vi "main.vi"() -> ()   [LabVIEW 2015]
uses:
  <vilib>/Utility/error.llb/whitespace.ctl
  <vilib>/MakerHub/LINX/Public/Peripherals/Analog/Analog Read N Chans.vi
  <vilib>/MakerHub/LINX/Public/Peripherals/Digital/Digital Write 1 Chan.vi
  <vilib>/MakerHub/LINX/Private/Local IO/LinxAnalogRead.vi
  <vilib>/MakerHub/LINX/Public/Utilities/Check Channel.vi
  <vilib>/MakerHub/LINX/Public/Peripherals/Digital/Digital Write N Chans.vi
  <vilib>/MakerHub/LINX/Private/Local IO/LinxDigitalWrite.vi
  <vilib>/Instr/_visa.llb/VISA Configure Serial Port (Instr).vi
  <vilib>/MakerHub/LINX/Public/Utilities/Open Serial.vi
  <vilib>/MakerHub/LINX/Private/Utilties/Generate Error.vi
  <vilib>/ptbypt/NI_PtbyPt.lvlib
  <vilib>/MakerHub/LINX/LMH-LINX.lvlib
  Report (lvlib)/Report - CSV/Report - CSV.lvlib
panel:
  out "baocao NG 2":bool
  out "baocao NG 1":bool
  in  "?":T1(tab)=enum."CONTROL & SUPERVISORY"
  in  "Result":i32(listbox)=-1
  in  "Delete table":bool
  out "Form QR ?":bool
  out "Data#":bool
  out "Found?":bool
  out "False Package":dbl
  out "SS3":bool=TRUE
  out "SS2":bool=TRUE
  out "SS1":bool=TRUE
  out "Processing Chart":cluster{dbl, dbl, dbl, dbl, "mean":dbl}(graph)={0.0, 0.0, 0.0, -16.408877733961745, "mean"=-16.408877733961745}
  out "WEIGHT PASS":bool
  out "Calculate\nValue":dbl=88.0
  out "DATA":string="ID: 3\nC/N: c8035\nQuantity: 42\nMass: 1.56\r\nS/N: 1\nC/N: vit dai\nQuantity: 3\nMass: 27\r\n"
  out "QR PASS":bool
  out "Well Package":i32
  out "Measurement\nValue":dbl format="%#.3f"
  in  "zero":bool
  in  "No. \nAccurate":dbl=10.0 format="%#_13g"
  in  "STOP":bool
  in  "Start measurement":bool caption="Manual\nMeasurement"
  out "CTHT1":bool=TRUE
  out "CTHT2":bool=TRUE
  out "Trigger1":bool
  out "Trigger 2":bool
  in  "k/lg bao bi":dbl=7.0 format="%#.3f"
  out "Run Loop":i32=6737
  out "?":T2(plugin-control)
  in  "measurement":dbl=38.0
  in  "calculate":dbl=50.0
  out "S/N":string
  out "C/N":string
  in  "Sensor Channels":u8[](array[numeric])=[0, 1, 2, 3, 4]
  in  "Path save data report":path=path "C:/Data"
  in  "COM Port Controller":refnum<visa-resource-name>="COM12"
  out "Quantity":i32=3
  out "Mass (kg):":dbl=27.0
  out "Tong K/lg (kg)":dbl=88.0
  in  "VISA resource name":refnum<visa-resource-name>="COM10"
  out "Data from HX711 box":i32[](array[numeric])
  out "size array":i32=233
  out "Raw data":dbl
  out "Fine Data":dbl=-16.408877733961745
  in  "zero":dbl=16.408877733961745
  in  "he so calib":dbl=8.552828494462736 format="%#_12g"
  in  "Low factor":cluster{"1":dbl, "2":dbl, "3":dbl}={"1"=177000.0, "2"=222000.0, "3"=-207250.0}
  in  "High Factor":cluster{"1":dbl, "2":dbl, "3":dbl}={"1"=1073000.0, "2"=1137000.0, "3"=703000.0} {"3" format="%#_15f"}
  in  "sample length":i32=100
  in  "No. model\nto Zero":i32=500
  in  "Pulse pin 2":u8=4
  in  "DIR pin 2":u8=3
  out "notifier out":refnum<notifier>
  in  "V-ref-trigger":dbl=0.2 format="%#_13g"
  out "Sensors Chart":T3(graph)={"Voltages[0]"=4.2626953125, "Voltages[1]"=4.27734375, "Voltages[2]"=4.2626953125, "Voltages[3]"=4.2626953125, "Voltages[4]"=4.2578125, "Voltages[5]"=0.0, "Voltages[6]"=0.0, "Voltages[7]"=0.0, "Voltages[8]"=0.0}
  in  "Enable pin 2":u8=2
  in  "Frequency (Hz) 2":u32=1600
  in  "Frequency (Hz)":u32=1600
  in  "Pulse pin":u8=4
  in  "DIR pin":u8=3
  in  "enable pin":u8=2
  in  "File name .csv":string="a"
  in  "Reset model":bool
  in  "button SS 1":bool
  in  "button SS 2":bool
  in  "button SS 3":bool
  in  "button CTHT 1":bool
  in  "button CTHT 2":bool
  out "STT":dbl format="%#_13g"
  out "gat hang 2":bool
  out "gat hang":bool
  out "Done QR":bool
  out "Appear":bool
  # "HÊò THÔìNG KIÊÒM TRA CHÂìT LÝÕòNG ÐOìNG GOìI THUÌNG HAÌNG\n THEO MAÞ QR & ÌKHÔìI LÝÕòNG"
  # "Table Result"
  # "(g)"
  # "(g)"
  # "Sensors"
  # "Control"
  # "Weight Transmit"
  # "Motor1"
  # "Motor2"
  # "Result Image Processing"
  # "Report"
  # "Distance Sensors and Limit Switch"
  # "TEST"
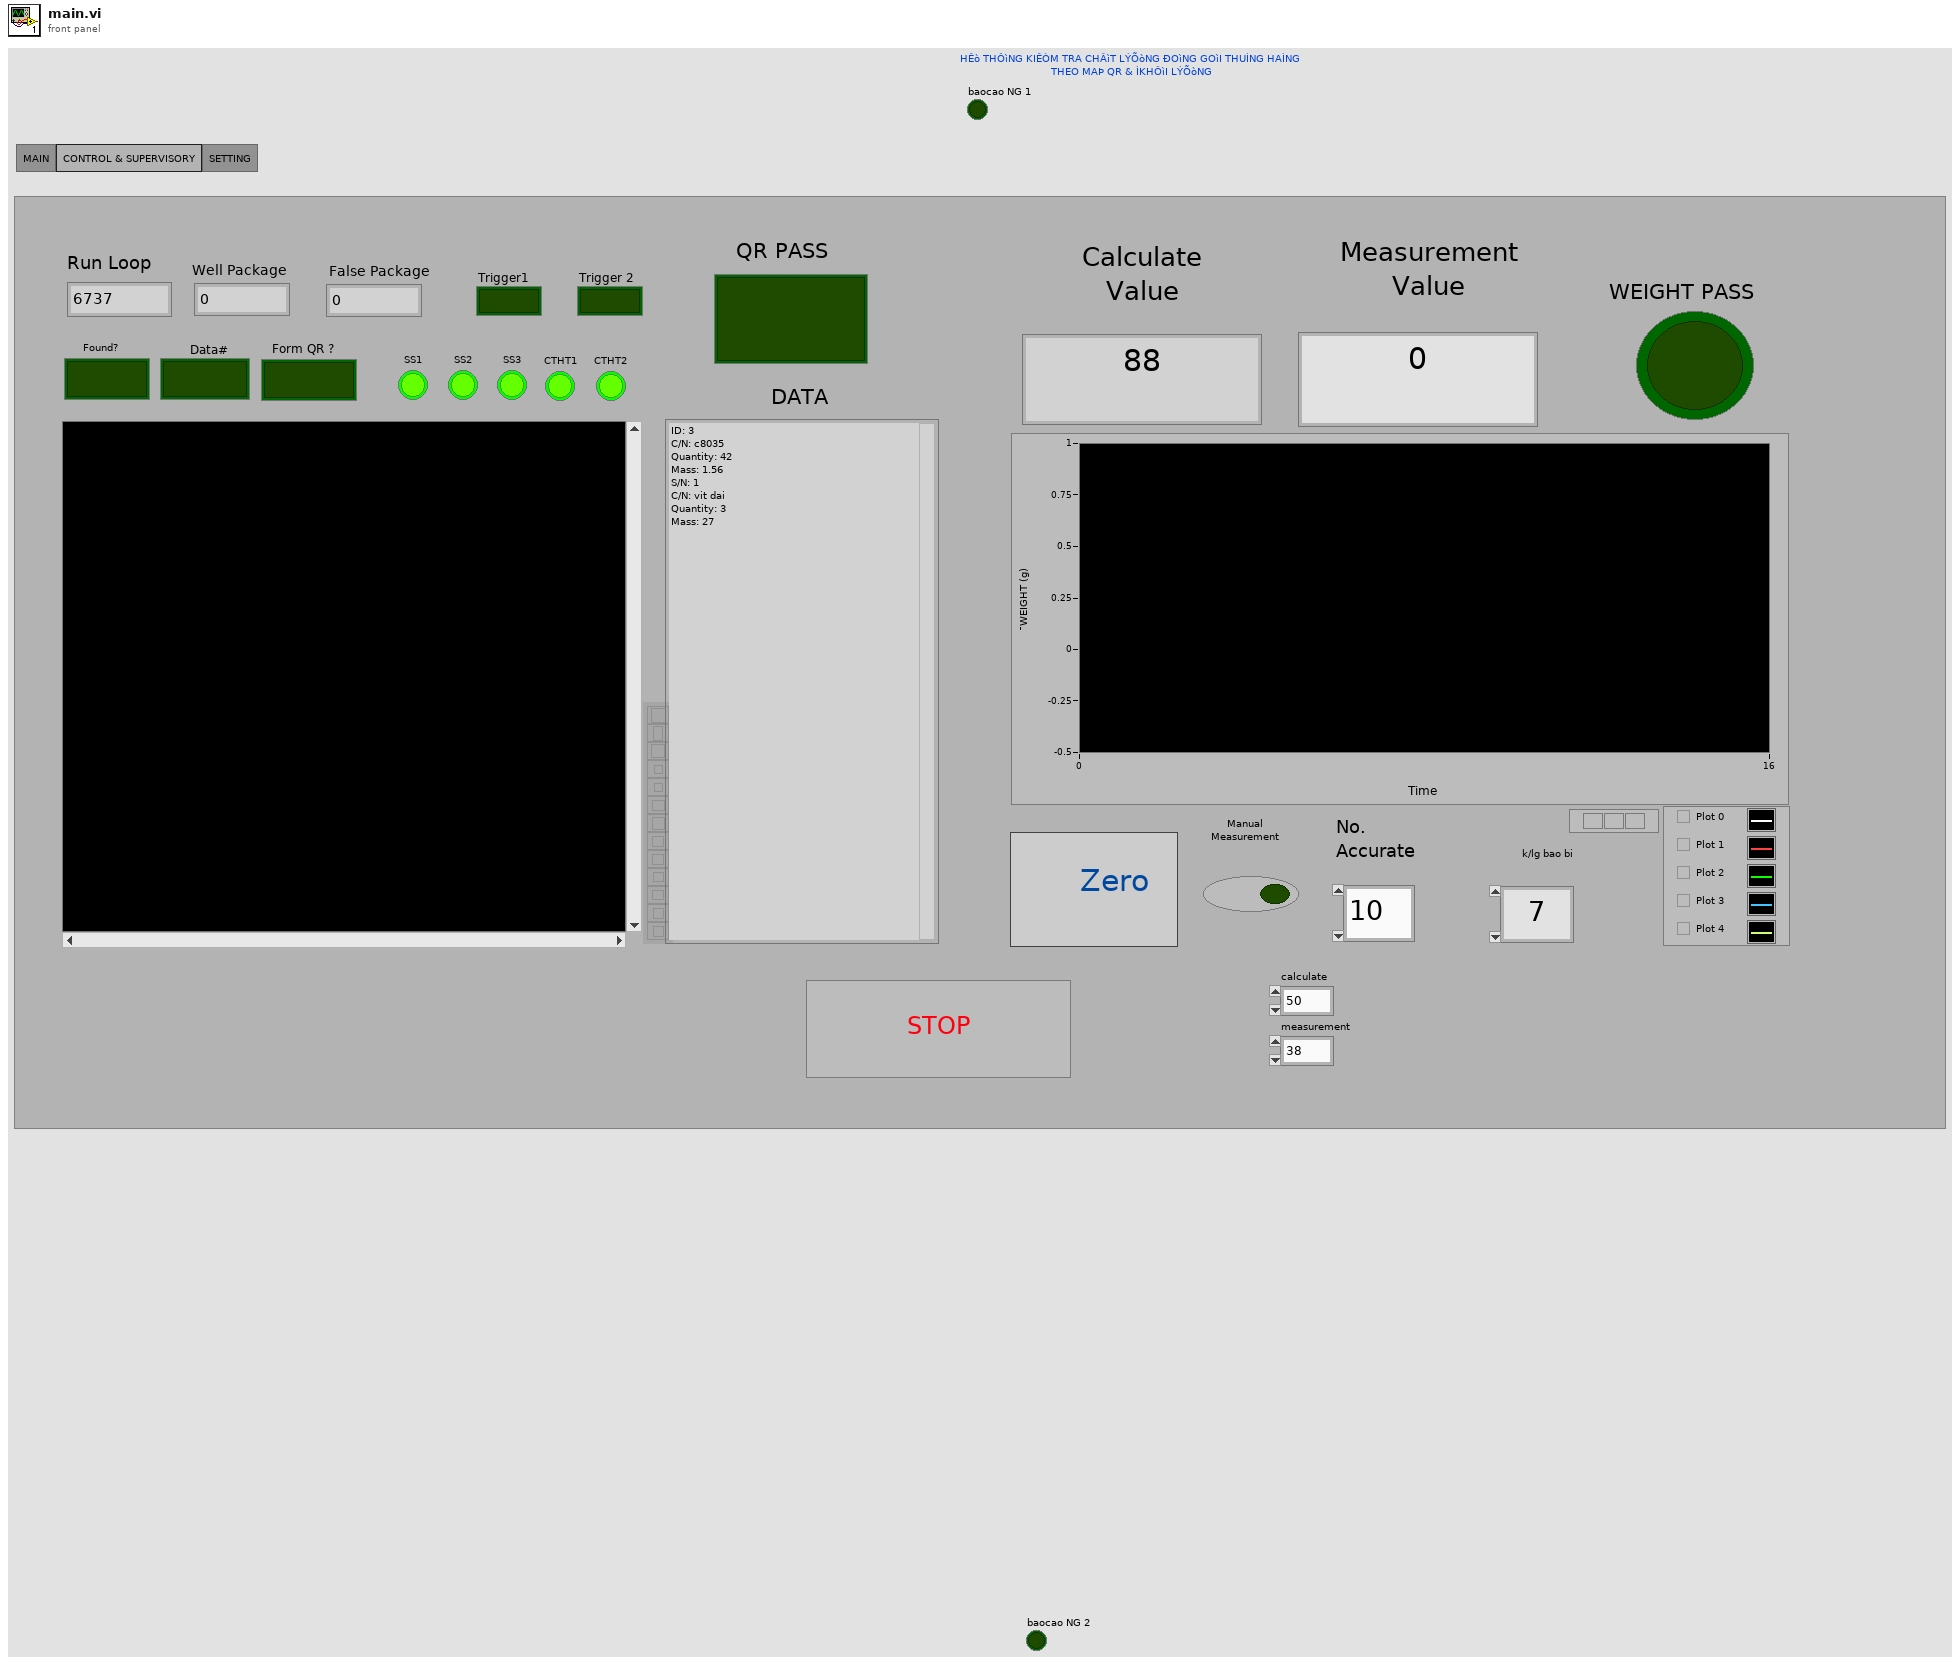
[diagram p1: front panel]
types:
  T1 = enum32{"MAIN", "CONTROL & SUPERVISORY", "SETTING"}
  T2 = typedef "IMAQ Image.ctl" = refnum<image>
  T3 = cluster{"Voltages[0]":dbl, "Voltages[1]":dbl, "Voltages[2]":dbl, "Voltages[3]":dbl, "Voltages[4]":dbl, "Voltages[5]":dbl, "Voltages[6]":dbl, "Voltages[7]":dbl, "Voltages[8]":dbl}
  T4 = cluster{"baud rate":u32, "data bits":u16, "parity":enum16{"None", "Odd", "Even", "Mark", "Space"}, "stop bits":u16, "flow control":u16}
  T5 = typedef "LMH-LINX.lvlib/LINX Ref.ctl" = cluster{"IO":T6, "Interface":T7, "LINX Device Config":T8}
  T6 = typedef "LMH-LINX.lvlib/Platform.ctl" = enum16{"Remote", "Local"}
  T7 = typedef "LMH-LINX.lvlib/Interface.ctl" = enum16{"Serial", "TCP"}
  T8 = typedef "LMH-LINX.lvlib/Device.lvlib/LINX Device Config.ctl" = cluster{"Interface":T7, "COM Port":refnum<visa-resource-name>, "TCP Configuration":T9, "Device Family":u8, "Device ID":u8, "Device Name":string, "TCP Ref":refnum<k5>, "Channels":T10}
  T9 = typedef "LMH-LINX.lvlib/Device.lvlib/TCP Config.ctl" = cluster{"IP Address":string, "Port":u16}
  T10 = typedef "LMH-LINX.lvlib/Channels.ctl" = cluster{"DI":u8[], "DO":u8[], "AI":u8[], "AO":u8[], "PWM":u8[], "QE":u8[], "UART":u8[], "I2C 2":u8[], "SPI":u8[], "CAN":u8[], "Servo":u8[], "AI Ref (V)":dbl, "AI Resolution (Bits)":u8, "AO Ref (V)":dbl, "AO Resolution (Bits)":u8}
  T11 = typedef "whitespace.ctl" = u16
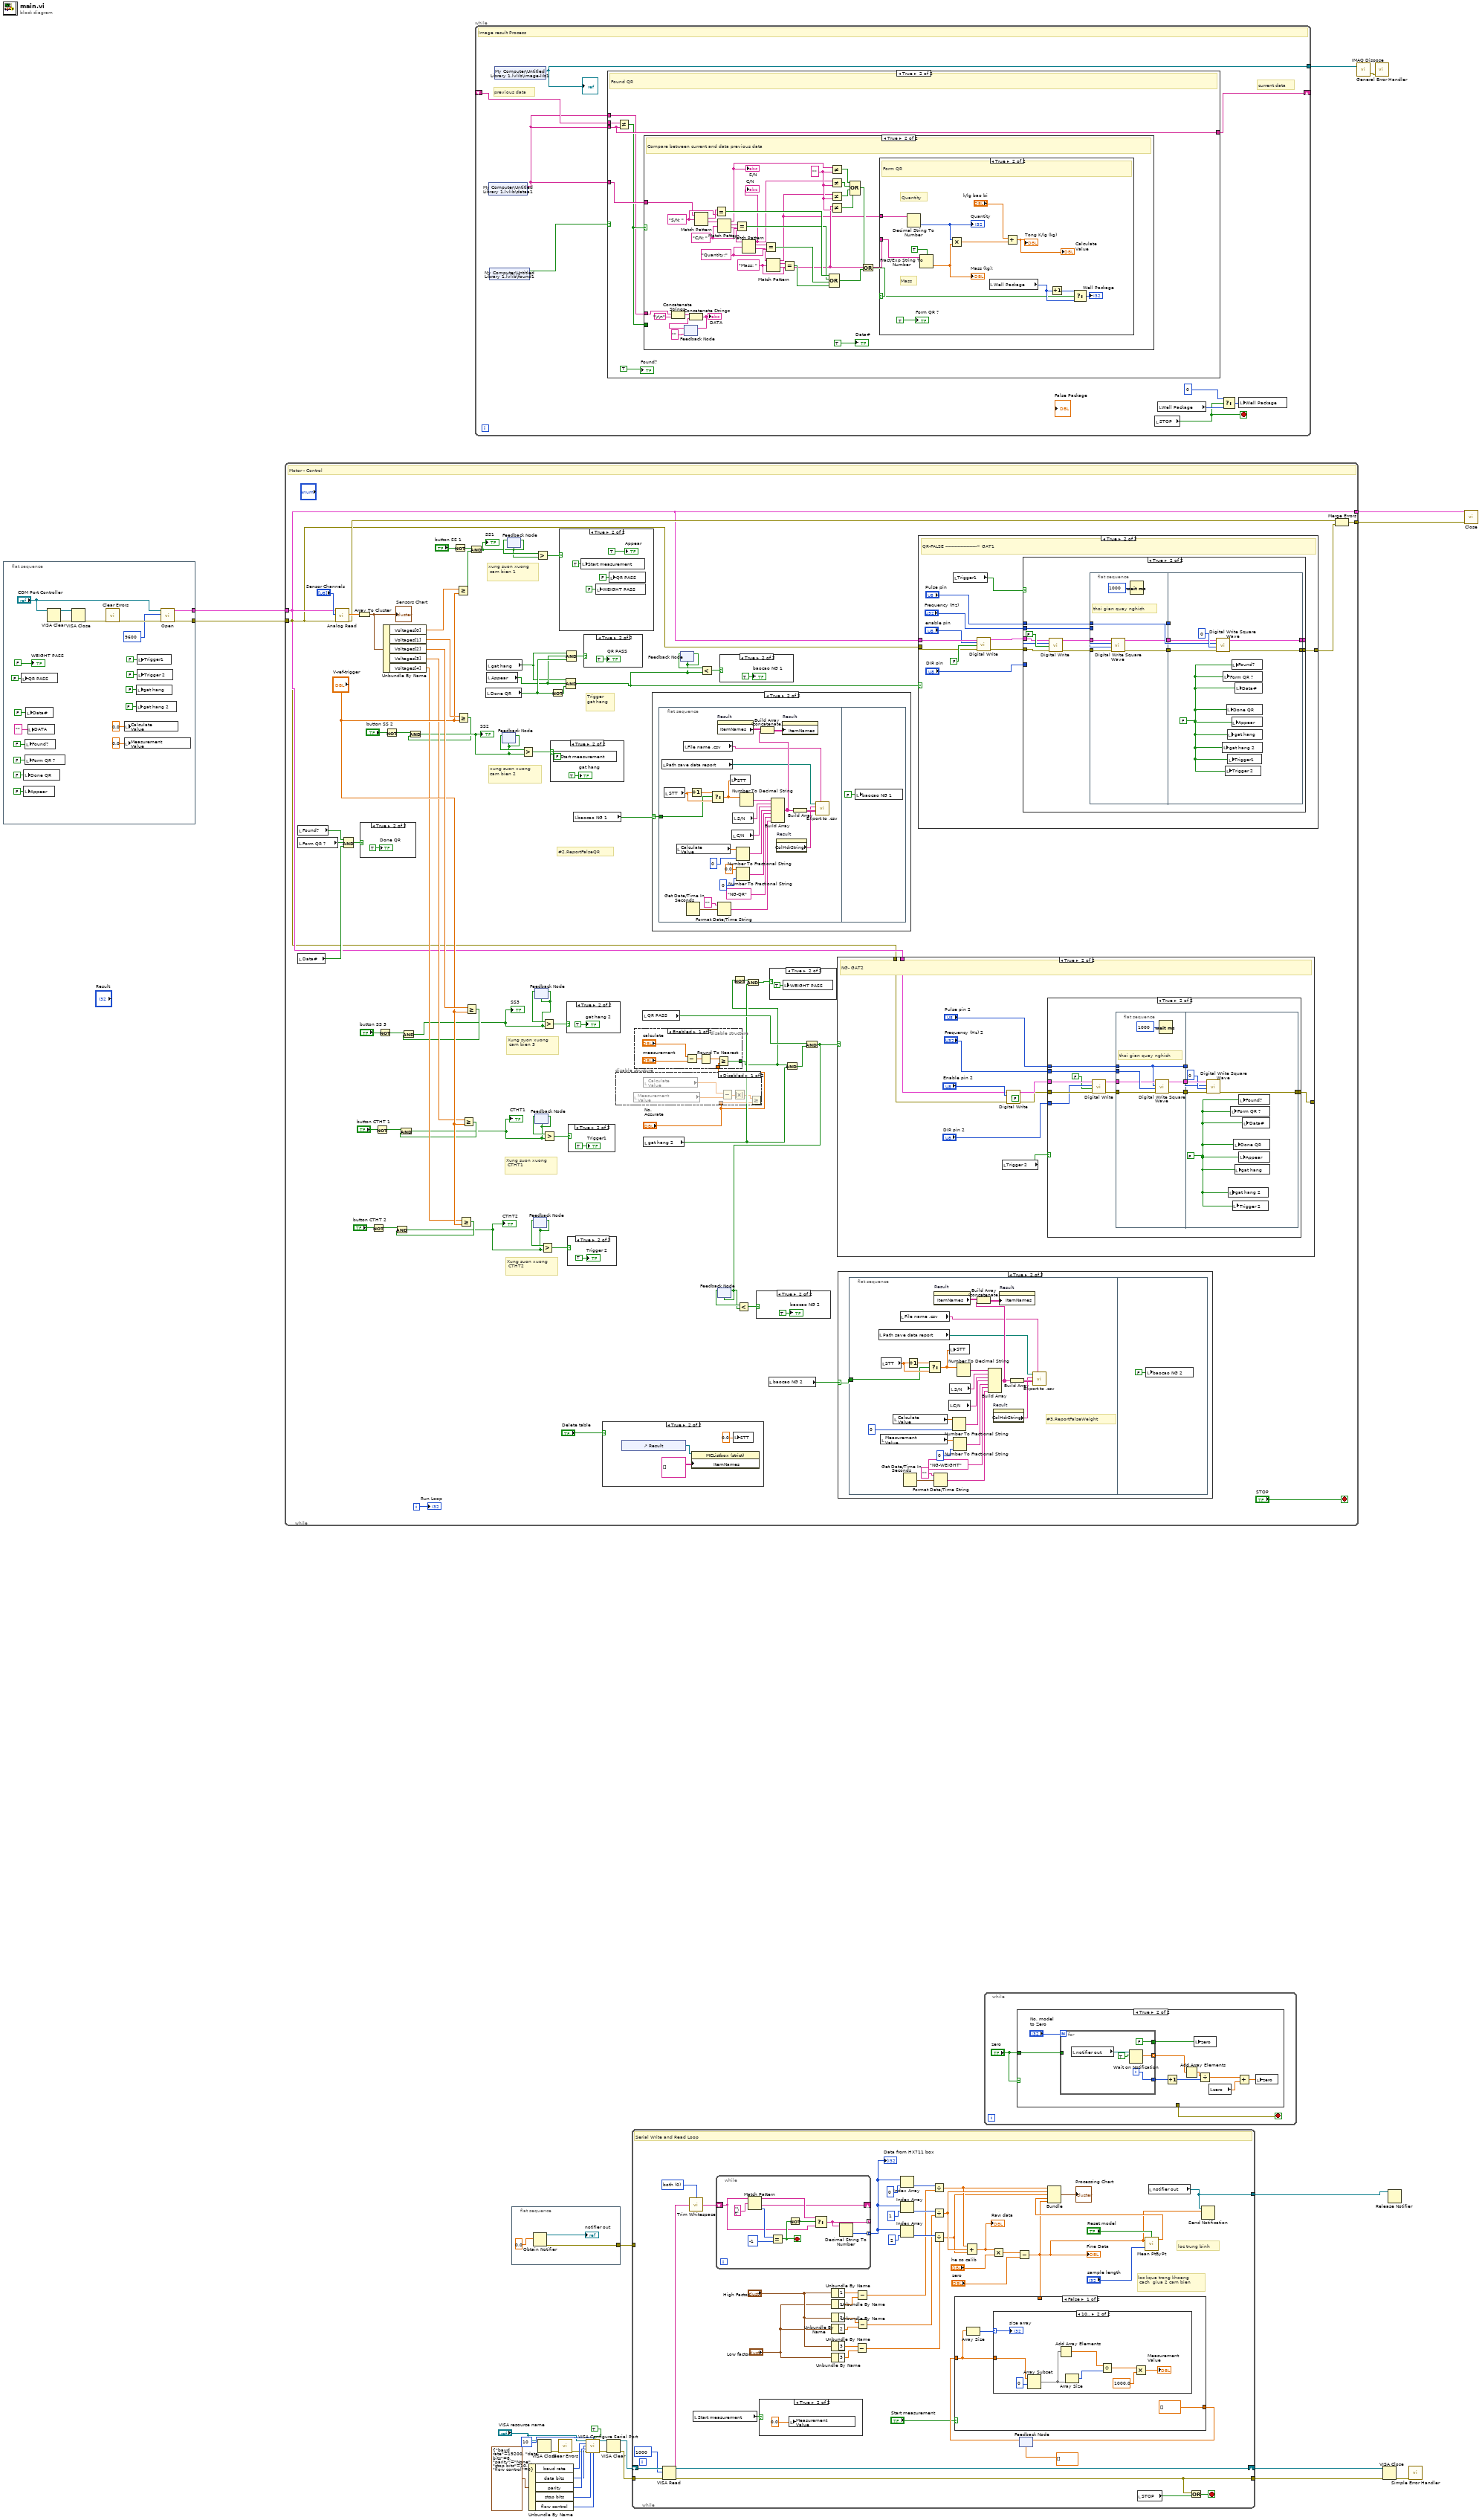
[diagram p0: block diagram]
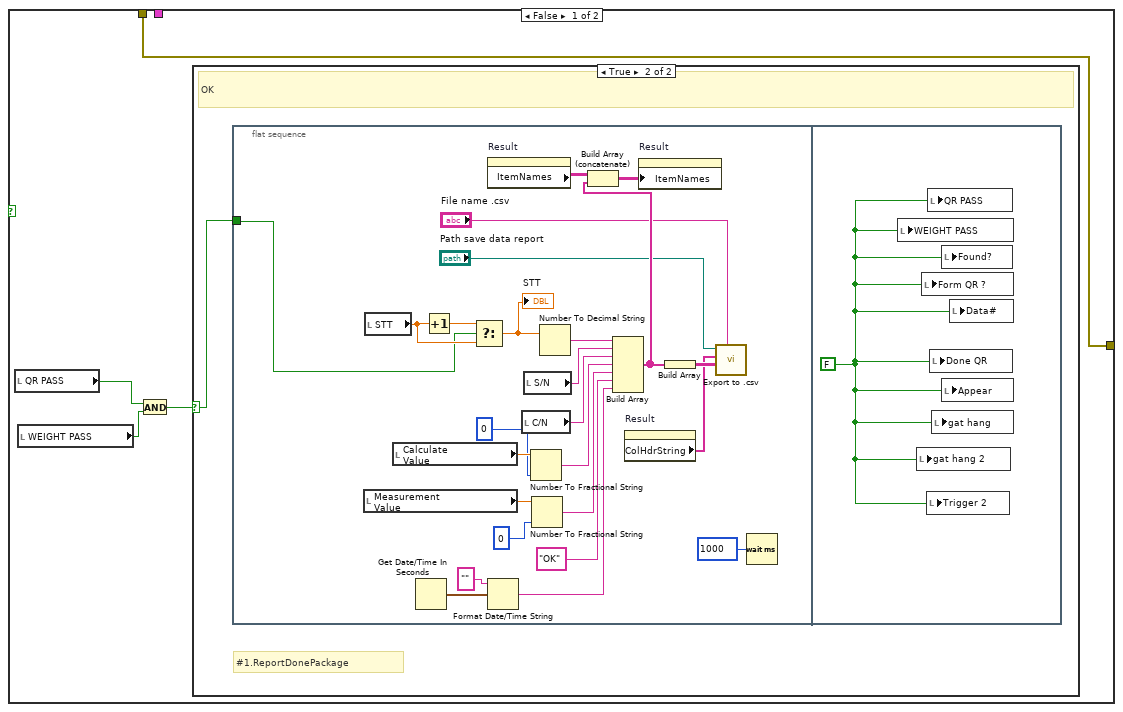
[diagram p15: hidden frame]
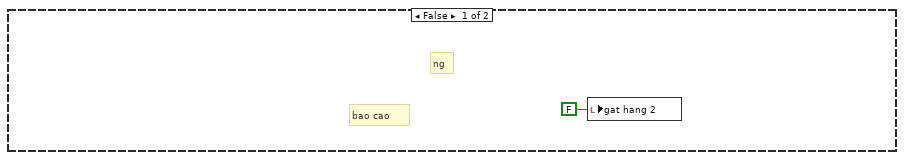
[diagram p16: hidden frame]
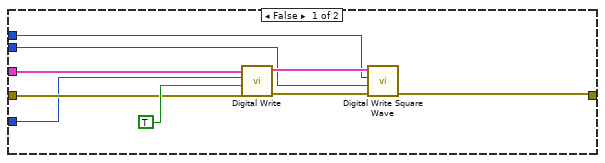
[diagram p17: hidden frame]
diagram:
  n1 = flat-sequence {
    tunnel: [w46] -> w2
    tunnel: [w45] -> w1
    frame #0 {
      n2 = local write "QR PASS"(FALSE ("QR PASS")) -> ()
      n3 = local write "Done QR"(FALSE ("Done QR")) -> ()
      n4 = local write "Appear"(FALSE ("Appear")) -> ()
      n5 = local write "Found?"(FALSE ("Form code ?")) -> ()
      n6 = local write "Form QR ?"(FALSE ("data current # data previous ?")) -> ()
      n7 = local write "Data#"(FALSE ("Found?")) -> ()
      n8 = local write "DATA"("" ("data-global")) -> ()
      n9 = VISA Clear(VISA resource name="COM Port Controller") -> (VISA resource name out=w43:refnum<visa-resource-name>, error out=w41:errorcluster)  [unwired: 1 in]
      n10 = VISA Close(VISA resource name=w43, error in (no error)=w41) -> (error out=w48:errorcluster)
      n11 = call <vilib>:"Clear Errors.vi"("error in (no error)"=w48) -> ("error out"=w47:errorcluster)  [unwired: 5 in, 1 out]
      n12 = local write "Calculate\nValue"(0.0 ("Calculated\nValue")) -> ()
      n13 = local write "Measurement\nValue"(0.0 ("Measurement\nValue")) -> ()
      n14 = local write "gat hang 2"(FALSE ("gat hang 2")) -> ()
      n15 = local write "gat hang"(FALSE ("gat hang")) -> ()
      n16 = local write "Trigger1"(FALSE ("Trigger1")) -> ()
      n17 = local write "Trigger 2"(FALSE ("Trigger 2")) -> ()
      n18 = call-poly <vilib>:"Open.vi"("Error In"=w47, "Baud Rate Override"=u32 9600, "Serial Port"="COM Port Controller") -> ("Error Out"=w45:errorcluster, "LINX Resource"=w46:T5)  [unwired: 6 in, 1 out]
      "WEIGHT PASS" <- FALSE ("WEIGHT PASS")
    }
  }
  n19 = while {
    tunnel: w2 -> [w65]
    tunnel: w1 -> [w64]
    tunnel: [w80] -> w4
    tunnel: [w65] -> w3
    i -> [w117]
    stop <- "STOP" stop-if-true
    # "#2.ReportFalseQR"
    # "Trigger\ngat hang"
    # "Xung suon xuong\n CTHT2"
    # "Xung suon xuong\n CTHT1"
    # "xung suon xuong\n cam bien 1"
    # "Xung suon xuong\n cam bien 3"
    # "xung suon xuong \ncam bien 2"
    # "Motor - Control"
    n20 = local read "Found?"() -> (w78:bool)
    n21 = local read "Form QR ?"() -> (w83:bool)
    n22 = local read "Data#"() -> (w84:bool)
    n23 = call-poly <vilib>:"Analog Read.vi"("Error In"=w64, "AI Channel(s)"="Sensor Channels", "LINX Resource"=w65) -> ("Error Out"=w79:errorcluster, "Voltages"=w119:dbl[])  [unwired: 5 in, 2 out]
    n24 = Compound Arithmetic op=AND(w78, w83, w84) -> (w72:bool)
    n25 = Array To Cluster(array=w119) -> (cluster=w109:T3)
    "Sensors Chart" <- w109
    n26 = case shown="True" w72 {
      frame False {
      }
      frame True {
        "Done QR" <- TRUE ("Done QR")
      }
    }
    n27 = Not(x="button CTHT 2") -> (.not. x?=w92:bool)
    n28 = Not(x="button CTHT 1") -> (.not. x?=w94:bool)
    n29 = Not(x="button SS 3") -> (.not. x?=w97:bool)
    n30 = Unbundle By Name(w109) -> ("Voltages[0]"=w115:dbl, "Voltages[1]"=w114:dbl, "Voltages[2]"=w113:dbl, "Voltages[3]"=w105:dbl, "Voltages[4]"=w104:dbl)
    n31 = Not(x="button SS 2") -> (.not. x?=w99:bool)
    n32 = Not(x="button SS 1") -> (.not. x?=w101:bool)
    n33 = Greater Or Equal?(x=w115, y="V-ref-trigger") -> (x >= y?=w103:bool)
    n34 = Greater Or Equal?(x=w114, y="V-ref-trigger") -> (x >= y?=w76:bool)
    n35 = And(x=w99, y=w76) -> (x .and. y?=w87:bool)
    "SS2" <- w87
    n36 = Greater Or Equal?(x=w104, y="V-ref-trigger") -> (x >= y?=w89:bool)
    n37 = And(x=w92, y=w89) -> (x .and. y?=w88:bool)
    "CTHT2" <- w88
    n38 = Greater Or Equal?(x=w105, y="V-ref-trigger") -> (x >= y?=w91:bool)
    n39 = And(x=w94, y=w91) -> (x .and. y?=w90:bool)
    "CTHT1" <- w90
    n40 = Greater Or Equal?(x=w113, y="V-ref-trigger") -> (x >= y?=w96:bool)
    n41 = And(x=w97, y=w96) -> (x .and. y?=w86:bool)
    "SS3" <- w86
    n42 = And(x=w101, y=w103) -> (x .and. y?=w75:bool)
    "SS1" <- w75
    n43 = local read "Done QR"() -> (w70:bool)
    n44 = local read "gat hang"() -> (w68:bool)
    n45 = local read "Appear"() -> (w69:bool)
    n46 = feedback #1(w87) -> (w118:bool)
    n47 = feedback-in #1(w87) -> ()
    n48 = feedback #2(w75) -> (w111:bool)
    n49 = feedback-in #2(w75) -> ()
    n50 = Greater?(x=w118, y=w87) -> (0:w74:bool)
    n51 = feedback #3(w88) -> (w107:bool)
    n52 = feedback-in #3(w88) -> ()
    n53 = feedback #4(w86) -> (w112:bool)
    n54 = feedback-in #4(w86) -> ()
    n55 = feedback #5(w90) -> (w108:bool)
    n56 = feedback-in #5(w90) -> ()
    n57 = Greater?(x=w111, y=w75) -> (0:w110:bool)
    n58 = Greater?(x=w107, y=w88) -> (0:w77:bool)
    n59 = Greater?(x=w112, y=w86) -> (0:w73:bool)
    n60 = Greater?(x=w108, y=w90) -> (0:w82:bool)
    n61 = case shown="True" w74 {
      frame False {
      }
      frame True {
        n62 = local write "Start measurement"(FALSE ("bat dau do")) -> ()
        "gat hang" <- TRUE ("gat hang")
      }
    }
    n63 = Not(x=w70) -> (.not. x?=w71:bool)
    n64 = case shown="True" w110 {
      frame False {
      }
      frame True {
        n65 = local write "Start measurement"(TRUE ("bat dau do")) -> ()
        n66 = local write "WEIGHT PASS"(FALSE ("WEIGHT PASS")) -> ()
        n67 = local write "QR PASS"(FALSE ("QR PASS")) -> ()
        "Appear" <- TRUE
      }
    }
    n68 = Compound Arithmetic op=AND(w68, w69, w71) -> (w54:bool)
    n69 = Compound Arithmetic op=AND(w68, w69, w70) -> (w67:bool)
    n70 = case shown="True" w73 {
      frame False {
      }
      frame True {
        "gat hang 2" <- TRUE ("gat hang 2")
      }
    }
    n71 = case shown="True" w77 {
      frame False {
      }
      frame True {
        "Trigger 2" <- TRUE ("Trigger 2")
      }
    }
    n72 = case shown="True" w82 {
      frame False {
      }
      frame True {
        "Trigger1" <- TRUE ("Trigger1")
      }
    }
    n73 = local read "baocao NG 1"() -> (w53:bool)
    n74 = case shown="True" w67 {
      frame False {
      }
      frame True {
        "QR PASS" <- TRUE ("QR PASS")
      }
    }
    n75 = case shown="True" "Delete table" {
      frame False {
      }
      frame True {
        n76 = control-ref of="Result"() -> (w175:refnum<vi>)
        n77 = property on="Property Node" class="MCListbox (strict)"(reference=w175, "ItemNames"=string[][] [] ("Item Names")) -> ()  [unwired: 1 in, 2 out]
        n78 = local write "STT"(0.0 ("STT")) -> ()
      }
    }
    n79 = disable-structure shown="Disabled" {
      disable-tunnel: "No. \nAccurate" -> [w177 _]
      frame Disabled {
        n80 = local read "Measurement\nValue"() -> (w179:dbl)
        n81 = local read "Calculate\nValue"() -> (w178:dbl)
        n82 = Subtract(x=w178, y=w179) -> (x-y=w180:dbl)
        n83 = Absolute Value(x=w180) -> (abs(x)=w181:dbl)
        n84 = Greater Or Equal?(x=w181, y=w177) -> ()  [unwired: 1 out]
      }
      frame Enabled {
      }
    }
    n85 = disable-structure shown="Enabled" {
      disable-tunnel: "No. \nAccurate" -> [w183 _]
      disable-tunnel: [w182 _] -> w58
      frame Enabled {
        n86 = Subtract(x="calculate", y="measurement") -> (x-y=w184:dbl)
        n87 = Round To Nearest(number=w184) -> (nearest integer value=w187:dbl)
        n88 = Greater Or Equal?(x=w187, y=w183) -> (x >= y?=w182:bool)
      }
      frame Disabled {
      }
    }
    n89 = local read "QR PASS"() -> (w63:bool)
    n90 = local read "gat hang 2"() -> (w60:bool)
    n91 = case shown="True" w53 {
      selector: w53 -> [_ w148]
      frame False {
      }
      frame True {
        n92 = flat-sequence {
          tunnel: w148 -> [w149]
          frame #0 {
            n93 = local read "Path save data report"() -> (w153:path)
            n94 = local read "STT"() -> (w166:dbl)
            n95 = local read "Calculate\nValue"() -> (w156:dbl)
            n96 = local read "File name .csv"() -> (w154:string)
            n97 = Get Date/Time In Seconds() -> (seconds since 1Jan1904=w170:timestamp)
            n98 = Increment(x=w166) -> (x+1=w165:dbl)
            n99 = Select(t=w165, s=w149, f=w166) -> (s? t:f=w151:dbl)
            n100 = property on="Result" class="MCListbox (strict)"() -> ("ItemNames"=w172:string[][])  [unwired: 2 in, 2 out]
            n101 = Format Date/Time String(time format string (%c)="", seconds (now)=w170) -> (date/time string=w160:string)  [unwired: 1 in]
            n102 = local write "STT"(w151) -> ()
            n103 = local read "C/N"() -> (w162:string)
            n104 = local read "S/N"() -> (w163:string)
            n105 = Number To Fractional String(number=w156, precision (6)=i16 0) -> (F-format string=w155:string)  [unwired: 2 in]
            n106 = Number To Fractional String(number=0.0, precision (6)=i16 0) -> (F-format string=w159:string)  [unwired: 2 in]
            n107 = Number To Decimal String(number=w151) -> (decimal integer string=w164:string)  [unwired: 1 in]
            n108 = Build Array(w164, w163, w162, w155, w159, "NG-QR" ("time format string (%c)"), w160) -> (w169:string[])
            n109 = Build Array (concatenate)(w172, w169) -> (w171:string[][])
            n110 = property on="Result" class="MCListbox (strict)"() -> ("ColHdrString"=w167:string[])  [unwired: 2 in, 2 out]
            n111 = property on="Result" class="MCListbox (strict)"("ItemNames"=w171) -> ()  [unwired: 2 in, 2 out]
            n112 = Build Array(w169) -> (w168:string[][])
            n113 = call "Export to .csv"("File name .csv"=w154, "Data - 2D"=w168, "ColHdrString - 1D"=w167, "Path in"=w153) -> ()  [unwired: 8 in]
          }
          frame #1 {
            n114 = local write "baocao NG 1"(FALSE ("baocao NG 1")) -> ()
          }
        }
      }
    }
    n115 = feedback #6(w54) -> (w56:bool)
    n116 = feedback-in #6(w54) -> ()
    n117 = Less?(x=w56, y=w54) -> (x < y?=w55:bool)
    n118 = case shown="True" w55 {
      frame False {
      }
      frame True {
        "baocao NG 1" <- TRUE ("baocao 1")
      }
    }
    n119 = Not(x=w58) -> (.not. x?=w61:bool)
    n120 = And(x=w61, y=w60) -> (x .and. y?=w62:bool)
    n121 = local read "baocao NG 2"() -> (w52:bool)
    n122 = case shown="True" w62 {
      frame False {
      }
      frame True {
        n123 = local write "WEIGHT PASS"(TRUE ("WEIGHT PASS")) -> ()
      }
    }
    n124 = And(x=w58, y=w60) -> (x .and. y?=w66:bool)
    n125 = And(x=w63, y=w66) -> (x .and. y?=w49:bool)
    n126 = feedback #7(w49) -> (w50:bool)
    n127 = feedback-in #7(w49) -> ()
    n128 = Less?(x=w50, y=w49) -> (x < y?=w51:bool)
    n129 = case shown="True" w51 {
      frame False {
      }
      frame True {
        "baocao NG 2" <- TRUE ("baocao 1")
      }
    }
    n130 = case shown="True" w49 {
      tunnel: [w194 w226] -> _
      tunnel: w65 -> [_ w224]
      tunnel: w64 -> [w194 w223]
      frame False {
        n131 = local read "QR PASS"() -> (w193:bool)
        n132 = local read "WEIGHT PASS"() -> (w192:bool)
        n133 = And(x=w193, y=w192) -> (x .and. y?=w191:bool)
        n134 = case shown="True" w191 {
          selector: w191 -> [_ w196]
          frame False {
            # "bao cao"
            # "ng"
            n135 = local write "gat hang 2"(FALSE ("WEIGHT PASS")) -> ()
          }
          frame True {
            # "#1.ReportDonePackage"
            # "OK"
            n136 = flat-sequence {
              tunnel: w196 -> [w197]
              frame #0 {
                n137 = local read "Measurement\nValue"() -> (w203:dbl)
                n138 = local read "STT"() -> (w213:dbl)
                n139 = local read "Calculate\nValue"() -> (w200:dbl)
                n140 = Get Date/Time In Seconds() -> (seconds since 1Jan1904=w218:timestamp)
                n141 = Increment(x=w213) -> (x+1=w212:dbl)
                n142 = Select(t=w212, s=w197, f=w213) -> (s? t:f=w211:dbl)
                "STT" <- w211
                n143 = property on="Result" class="MCListbox (strict)"() -> ("ItemNames"=w220:string[][])  [unwired: 2 in, 2 out]
                n144 = Format Date/Time String(time format string (%c)="", seconds (now)=w218) -> (date/time string=w205:string)  [unwired: 1 in]
                n145 = local read "C/N"() -> (w207:string)
                n146 = local read "S/N"() -> (w208:string)
                n147 = Number To Fractional String(number=w200, precision (6)=i16 0) -> (F-format string=w199:string)  [unwired: 2 in]
                n148 = Number To Fractional String(number=w203, precision (6)=i16 0) -> (F-format string=w204:string)  [unwired: 2 in]
                n149 = Number To Decimal String(number=w211) -> (decimal integer string=w210:string)  [unwired: 1 in]
                n150 = Build Array(w210, w208, w207, w199, w204, "OK" ("time format string (%c)"), w205) -> (w217:string[])
                n151 = Build Array (concatenate)(w220, w217) -> (w219:string[][])
                n152 = property on="Result" class="MCListbox (strict)"() -> ("ColHdrString"=w215:string[])  [unwired: 2 in, 2 out]
                n153 = property on="Result" class="MCListbox (strict)"("ItemNames"=w219) -> ()  [unwired: 2 in, 2 out]
                n154 = Build Array(w217) -> (w216:string[][])
                n155 = call "Export to .csv"("File name .csv"="File name .csv", "Data - 2D"=w216, "ColHdrString - 1D"=w215, "Path in"="Path save data report") -> ()  [unwired: 8 in]
                n156 = Wait (ms)(milliseconds to wait=u32 1000) -> ()  [unwired: 1 out]
              }
              frame #1 {
                w222 = FALSE ("WEIGHT PASS")
                n157 = local write "WEIGHT PASS"(w222) -> ()
                n158 = local write "gat hang 2"(w222) -> ()
                n159 = local write "Form QR ?"(w222) -> ()
                n160 = local write "Trigger 2"(w222) -> ()
                n161 = local write "QR PASS"(w222) -> ()
                n162 = local write "Done QR"(w222) -> ()
                n163 = local write "gat hang"(w222) -> ()
                n164 = local write "Found?"(w222) -> ()
                n165 = local write "Appear"(w222) -> ()
                n166 = local write "Data#"(w222) -> ()
              }
            }
          }
        }
      }
      frame True {
        # "NG- GAT2"
        n167 = local read "Trigger 2"() -> (w225:bool)
        n168 = call-poly <vilib>:"Digital Write.vi"("Error In"=w223, "Output Value"=FALSE, "DO Channel"="Enable pin 2", "LINX Resource"=w224) -> ("Error Out"=w227:errorcluster, "LINX Resource"=w228:T5)  [unwired: 6 in]
        n169 = case shown="True" w225 {
          tunnel: "Pulse pin 2" -> [w237 w254]
          tunnel: "DIR pin 2" -> [w235 w250]
          tunnel: "Frequency (Hz) 2" -> [w236 w253]
          tunnel: w228 -> [w239 w252]
          tunnel: w227 -> [w238 w251]
          tunnel: [w234 w244] -> w226
          frame False {
            n170 = call-poly <vilib>:"Digital Write.vi"("Error In"=w238, "Output Value"=TRUE, "DO Channel"=w235, "LINX Resource"=w239) -> ("Error Out"=w241:errorcluster, "LINX Resource"=w240:T5)  [unwired: 6 in]
            n171 = call <vilib>:"Digital Write Square Wave.vi"("Error In"=w241, "Frequency (Hz)"=w236, "Channel"=w237, "LINX Resource"=w240) -> ("Error Out"=w234:errorcluster)  [unwired: 6 in, 1 out]
          }
          frame True {
            n172 = call-poly <vilib>:"Digital Write.vi"("Error In"=w251, "Output Value"=FALSE, "DO Channel"=w250, "LINX Resource"=w252) -> ("Error Out"=w248:errorcluster, "LINX Resource"=w249:T5)  [unwired: 6 in]
            n173 = flat-sequence {
              tunnel: w254 -> [w255]
              tunnel: w253 -> [w260]
              tunnel: w249 -> [w259]
              tunnel: w248 -> [w258]
              tunnel: [w257] -> w247
              tunnel: [w256] -> w246
              tunnel: [w255] -> w245
              tunnel: w247 -> [w267]
              tunnel: w246 -> [w266]
              tunnel: w245 -> [w264]
              tunnel: [w263] -> w244
              frame #0 {
                # "thoi gian quay nghich"
                n174 = call <vilib>:"Digital Write Square Wave.vi"("Error In"=w258, "Frequency (Hz)"=w260, "Channel"=w255, "LINX Resource"=w259) -> ("Error Out"=w256:errorcluster, "LINX Resource"=w257:T5)  [unwired: 6 in]
                n175 = Wait (ms)(milliseconds to wait=u32 1000) -> ()  [unwired: 1 out]
              }
              frame #1 {
                w262 = FALSE ("WEIGHT PASS")
                n176 = call <vilib>:"Digital Write Square Wave.vi"("Error In"=w266, "Frequency (Hz)"=u32 0, "Channel"=w264, "LINX Resource"=w267) -> ("Error Out"=w263:errorcluster)  [unwired: 6 in, 1 out]
                n177 = local write "gat hang 2"(w262) -> ()
                n178 = local write "Form QR ?"(w262) -> ()
                n179 = local write "Trigger 2"(w262) -> ()
                n180 = local write "Done QR"(w262) -> ()
                n181 = local write "gat hang"(w262) -> ()
                n182 = local write "Found?"(w262) -> ()
                n183 = local write "Appear"(w262) -> ()
                n184 = local write "Data#"(w262) -> ()
              }
            }
          }
        }
      }
    }
    n185 = case shown="True" w52 {
      selector: w52 -> [_ w121]
      frame False {
      }
      frame True {
        n186 = flat-sequence {
          tunnel: w121 -> [w122]
          frame #0 {
            # "#3.ReportFalseWeight"
            n187 = local read "Path save data report"() -> (w125:path)
            n188 = local read "Measurement\nValue"() -> (w131:dbl)
            n189 = local read "STT"() -> (w139:dbl)
            n190 = local read "Calculate\nValue"() -> (w128:dbl)
            n191 = local read "File name .csv"() -> (w126:string)
            n192 = Get Date/Time In Seconds() -> (seconds since 1Jan1904=w143:timestamp)
            n193 = Increment(x=w139) -> (x+1=w138:dbl)
            n194 = Select(t=w138, s=w122, f=w139) -> (s? t:f=w124:dbl)
            n195 = property on="Result" class="MCListbox (strict)"() -> ("ItemNames"=w145:string[][])  [unwired: 2 in, 2 out]
            n196 = Format Date/Time String(time format string (%c)="", seconds (now)=w143) -> (date/time string=w133:string)  [unwired: 1 in]
            n197 = local read "C/N"() -> (w135:string)
            n198 = local write "STT"(w124) -> ()
            n199 = local read "S/N"() -> (w136:string)
            n200 = Number To Fractional String(number=w128, precision (6)=i16 0) -> (F-format string=w127:string)  [unwired: 2 in]
            n201 = Number To Fractional String(number=w131, precision (6)=i16 0) -> (F-format string=w132:string)  [unwired: 2 in]
            n202 = Number To Decimal String(number=w124) -> (decimal integer string=w137:string)  [unwired: 1 in]
            n203 = Build Array(w137, w136, w135, w127, w132, "NG-WEIGHT" ("time format string (%c)"), w133) -> (w142:string[])
            n204 = Build Array (concatenate)(w145, w142) -> (w144:string[][])
            n205 = property on="Result" class="MCListbox (strict)"() -> ("ColHdrString"=w140:string[])  [unwired: 2 in, 2 out]
            n206 = property on="Result" class="MCListbox (strict)"("ItemNames"=w144) -> ()  [unwired: 2 in, 2 out]
            n207 = Build Array(w142) -> (w141:string[][])
            n208 = call "Export to .csv"("File name .csv"=w126, "Data - 2D"=w141, "ColHdrString - 1D"=w140, "Path in"=w125) -> ()  [unwired: 8 in]
          }
          frame #1 {
            n209 = local write "baocao NG 2"(FALSE ("baocao NG 2")) -> ()
          }
        }
      }
    }
    n210 = case shown="True" w54 {
      tunnel: w65 -> [_ w279]
      tunnel: w64 -> [w271 w278]
      tunnel: [w271 w277] -> w81
      frame False {
        # "PASS QR ---------> CHECK WEIGHT"
      }
      frame True {
        # "QR-FALSE ---------------------> GAT1"
        n211 = local read "Trigger1"() -> (w276:bool)
        n212 = call-poly <vilib>:"Digital Write.vi"("Error In"=w278, "Output Value"=FALSE, "DO Channel"="enable pin", "LINX Resource"=w279) -> ("Error Out"=w280:errorcluster, "LINX Resource"=w281:T5)  [unwired: 6 in]
        n213 = case shown="True" w276 {
          tunnel: w281 -> [w292 w302]
          tunnel: w280 -> [w291 w301]
          tunnel: "DIR pin" -> [w290 w300]
          tunnel: [w289 w299] -> _
          tunnel: [w288 w298] -> w277
          tunnel: "Pulse pin" -> [w284 w295]
          tunnel: "Frequency (Hz)" -> [w283 w293]
          frame False {
            n214 = call-poly <vilib>:"Digital Write.vi"("Error In"=w291, "Output Value"=TRUE, "DO Channel"=w290, "LINX Resource"=w292) -> ("Error Out"=w286:errorcluster, "LINX Resource"=w285:T5)  [unwired: 6 in]
            n215 = call <vilib>:"Digital Write Square Wave.vi"("Error In"=w286, "Frequency (Hz)"=w283, "Channel"=w284, "LINX Resource"=w285) -> ("Error Out"=w288:errorcluster, "LINX Resource"=w289:T5)  [unwired: 6 in]
          }
          frame True {
            n216 = call-poly <vilib>:"Digital Write.vi"("Error In"=w301, "Output Value"=FALSE, "DO Channel"=w300, "LINX Resource"=w302) -> ("Error Out"=w304:errorcluster, "LINX Resource"=w303:T5)  [unwired: 6 in]
            n217 = flat-sequence {
              tunnel: w304 -> [w312]
              tunnel: w303 -> [w311]
              tunnel: [w310] -> w297
              tunnel: [w309] -> w296
              tunnel: w295 -> [w307]
              tunnel: [w307] -> w294
              tunnel: w293 -> [w306]
              tunnel: [w315] -> w298
              tunnel: [w316] -> w299
              tunnel: w297 -> [w318]
              tunnel: w296 -> [w317]
              tunnel: w294 -> [w314]
              frame #0 {
                # "thoi gian quay nghich"
                n218 = call <vilib>:"Digital Write Square Wave.vi"("Error In"=w312, "Frequency (Hz)"=w306, "Channel"=w307, "LINX Resource"=w311) -> ("Error Out"=w309:errorcluster, "LINX Resource"=w310:T5)  [unwired: 6 in]
                n219 = Wait (ms)(milliseconds to wait=u32 1000) -> ()  [unwired: 1 out]
              }
              frame #1 {
                w313 = FALSE ("WEIGHT PASS")
                n220 = call <vilib>:"Digital Write Square Wave.vi"("Error In"=w317, "Frequency (Hz)"=u32 0, "Channel"=w314, "LINX Resource"=w318) -> ("Error Out"=w315:errorcluster, "LINX Resource"=w316:T5)  [unwired: 6 in]
                n221 = local write "gat hang 2"(w313) -> ()
                n222 = local write "Form QR ?"(w313) -> ()
                n223 = local write "Trigger 2"(w313) -> ()
                n224 = local write "Done QR"(w313) -> ()
                n225 = local write "gat hang"(w313) -> ()
                n226 = local write "Trigger1"(w313) -> ()
                n227 = local write "Found?"(w313) -> ()
                n228 = local write "Appear"(w313) -> ()
                n229 = local write "Data#"(w313) -> ()
              }
            }
          }
        }
      }
    }
    n230 = Merge Errors(w79, w81) -> (w80:errorcluster)
    "Run Loop" <- w117
  }
  n231 = while {
    shift-right: [w330] -> _
    shift-left: _ -> [w329]
    tunnel: [w326] -> w5
    stop <- w331 stop-if-true
    # "previous data"
    # "current data"
    # "Image result Process"
    n232 = shared-variable "My Computer\\Untitled Library 1.lvlib\\dataa1"() -> (w327:string)  [unwired: 1 in, 1 out]
    n233 = shared-variable "My Computer\\Untitled Library 1.lvlib\\found1"() -> (w328:bool)  [unwired: 1 in, 1 out]
    n234 = shared-variable "My Computer\\Untitled Library 1.lvlib\\image-lib1"() -> (w326:refnum<image>)  [unwired: 1 in, 1 out]
    "?" <- w326
    n235 = case shown="True" w328 {
      tunnel: w327 -> [_ w339]
      tunnel: [w335 w340] -> w330
      tunnel: w329 -> [w335 w341]
      tunnel: w327 -> [_ w340]
      tunnel: w327 -> [_ w336]
      frame False {
        # "Found QR"
      }
      frame True {
        # "Found QR"
        n236 = Not Equal?(x=w341, y=w340) -> (x != y?=w337:bool)
        n237 = case shown="True" w337 {
          tunnel: w339 -> [_ w345]
          tunnel: w337 -> [_ _]
          tunnel: w336 -> [_ w359]
          frame False {
          }
          frame True {
            w367 = "" ("y")
            w352 = "C/N: " ("regular expression")
            w353 = "S/N: " ("regular expression")
            w350 = "Mass: " ("regular expression")
            w351 = "Quantity:" ("regular expression")
            # "Compare between current and data previous data"
            n238 = Concatenate Strings(w359, "\r\n" ("End of Line Constant")) -> (w356:string)
            n239 = feedback #8("") -> (w355:string)
            n240 = Concatenate Strings(w356, w355) -> (w354:string)
            "DATA" <- w354
            n241 = feedback-in #8(w354) -> ()
            n242 = Match Pattern(string=w345, regular expression=w353) -> (match substring=w373:string, after substring=w348:string)  [unwired: 1 in, 2 out]
            n243 = Equal?(x=w373, y=w353) -> (x = y?=w372:bool)
            n244 = Match Pattern(string=w348, regular expression=w352) -> (before substring=w344:string, match substring=w374:string, after substring=w347:string)  [unwired: 1 in, 1 out]
            "S/N" <- w344
            n245 = Equal?(x=w374, y=w352) -> (x = y?=w371:bool)
            n246 = Match Pattern(string=w347, regular expression=w351) -> (before substring=w343:string, match substring=w375:string, after substring=w346:string)  [unwired: 1 in, 1 out]
            "C/N" <- w343
            n247 = Equal?(x=w375, y=w351) -> (x = y?=w370:bool)
            n248 = Match Pattern(string=w346, regular expression=w350) -> (before substring=w342:string, match substring=w376:string, after substring=w349:string)  [unwired: 1 in, 1 out]
            n249 = Equal?(x=w376, y=w350) -> (x = y?=w369:bool)
            n250 = Compound Arithmetic op=OR(w372, w371, w370, w369) -> (w362:bool)
            n251 = Not Equal?(x=w344, y=w367) -> (x != y?=w366:bool)
            n252 = Not Equal?(x=w343, y=w367) -> (x != y?=w365:bool)
            n253 = Not Equal?(x=w342, y=w367) -> (x != y?=w364:bool)
            n254 = Not Equal?(x=w349, y=w367) -> (x != y?=w363:bool)
            n255 = Compound Arithmetic op=OR(w366, w365, w364, w363) -> (w361:bool)
            n256 = Compound Arithmetic op=OR(w361, w362) -> (w360:bool)
            n257 = case shown="True" w360 {
              selector: w360 -> [_ w382]
              tunnel: w342 -> [_ w383]
              tunnel: w349 -> [_ w380]
              frame False {
              }
              frame True {
                # "Mass"
                # "Quantity"
                # "Form QR"
                n258 = Decimal String To Number(string=w383) -> (number=w385:i32)  [unwired: 2 in, 1 out]
                "Quantity" <- w385
                n259 = Fract/Exp String To Number(use system decimal point (T)=TRUE, string=w380) -> (number=w384:dbl)  [unwired: 2 in, 1 out]
                "Mass (kg):" <- w384
                n260 = Multiply(x=w385, y=w384) -> (x*y=w377:dbl)
                n261 = local read "Well Package"() -> (w388:i32)
                n262 = Add(x="k/lg bao bi", y=w377) -> (x+y=→"Tong K/lg (kg)" →"Calculate\nValue":dbl)
                n263 = Increment(x=w388) -> (x+1=w387:i32)
                n264 = Select(t=w387, s=w382, f=w388) -> (s? t:f=→"Well Package":i32)
                "Form QR ?" <- TRUE ("Form code ?")
              }
            }
            "Data#" <- TRUE ("data current # data previous ?")
          }
        }
        "Found?" <- TRUE ("Found?")
      }
    }
    n265 = local read "STOP"() -> (w331:bool)
    n266 = local read "Well Package"() -> (w332:i32)
    n267 = Select(t=0, s=w331, f=w332) -> (s? t:f=w334:i32)
    n268 = local write "Well Package"(w334) -> ()
  }
  n269 = flat-sequence {
    tunnel: [w390] -> w8
    frame #0 {
      n270 = Obtain Notifier(notification data type=0.0 ("Y Scale.Range:Maximum")) -> (notifier out=→"notifier out":refnum<notifier>, error out=w390:errorcluster)  [unwired: 3 in, 1 out]
    }
  }
  n271 = Unbundle By Name(T4 {"baud rate"=19200, "data bits"=8, "parity"=enum."None", "stop bits"=10, "flow control"=0} ("Serial Settings")) -> ("baud rate"=w23:u32, "data bits"=w24:u16, "parity"=w25:enum16{"None", "Odd", "Even", "Mark", "Space"}, "stop bits"=w26:u16, "flow control"=w17:u16)
  n272 = VISA Close(VISA resource name="VISA resource name") -> (error out=w13:errorcluster)  [unwired: 1 in]
  n273 = call <vilib>:"Clear Errors.vi"("error in (no error)"=w13) -> ("error out"=w12:errorcluster)  [unwired: 5 in, 1 out]
  n274 = call-poly "VISA Configure Serial Port"("VISA resource name"="VISA resource name", "termination char\n(0xA = '\\n' = LF)"=u8 10 ("Termination Character"), "Enable Termination\nChar (T)"=TRUE ("End Read on\n Termination Character?"), "baud rate (9600)"=w23, "data bits (8)"=w24, "parity (0:none)"=w25, "error in (no error)"=w12, "stop bits (10: 1 bit)"=w26, "flow control (0:none)"=w17) -> ("VISA resource name out"=w16:refnum<visa-resource-name>, "error out"=w10:errorcluster)  [unwired: 1 in, 4 out]
  n275 = VISA Clear(VISA resource name=w16, error in (no error)=w10) -> (VISA resource name out=w11:refnum<visa-resource-name>, error out=w9:errorcluster)
  n276 = while {
    shift-right: [w438] -> w18
    shift-left: w11 -> [w437]
    tunnel: w9 -> [w436]
    tunnel: [w435] -> w19
    tunnel: w8 -> [_]
    tunnel: [w397] -> w7
    stop <- w413 stop-if-true
    w433 = T11 0 items=["both", "start of string", "end of string"] ("location (both)")
    # "loc kqua trong khoang\n cach  giua 2 cam bien"
    # "loc trung binh"
    # "Serial Write and Read Loop"
    n277 = VISA Read(VISA resource name=w437, byte count=u32 1000 ("Read Count"), error in (no error)=w436) -> (VISA resource name out=w438:refnum<visa-resource-name>, read buffer=w417:string, error out=w435:errorcluster)  [unwired: 1 out]
    n278 = call <vilib>:"Trim Whitespace.vi"("string"=w417, "location (both)"=w433) -> ("trimmed string"=w432:string)
    n279 = local read "Start measurement"() -> (w400:bool)
    n280 = while {
      shift-right: [w459] -> _
      shift-left: w432 -> [w456]
      tunnel: [w458] -> _ mode=indexing
      tunnel: [w455] -> w418 mode=indexing
      stop <- w462 stop-if-true
      n281 = Match Pattern(string=w456, regular expression="\t") -> (before substring=w460:string, after substring=w459:string, offset past match=w464:i32)  [unwired: 1 in, 1 out]
      n282 = Equal?(x=w464, y=-1) -> (x = y?=w462:bool)
      n283 = Not(x=w462) -> (.not. x?=w461:bool)
      n284 = Select(t=w460, s=w461, f=w456) -> (s? t:f=w458:string)
      n285 = Decimal String To Number(string=w458) -> (number=w455:i32)  [unwired: 2 in, 1 out]
    }
    "Data from HX711 box" <- w418
    n286 = case shown="True" w400 {
      frame False {
      }
      frame True {
        n287 = local write "Measurement\nValue"(0.0 ("x/y")) -> ()
      }
    }
    n288 = Unbundle By Name "Unbundle By Name"("High Factor") -> ("1"=w412:dbl)
    n289 = Unbundle By Name("Low factor") -> ("1"=w411:dbl)
    n290 = Unbundle By Name("High Factor") -> ("2"=w409:dbl)
    n291 = Unbundle By Name("Low factor") -> ("2"=w410:dbl)
    n292 = Unbundle By Name("High Factor") -> ("3"=w408:dbl)
    n293 = Unbundle By Name("Low factor") -> ("3"=w407:dbl)
    n294 = Subtract(x=w408, y=w407) -> (x-y=w403:dbl)
    n295 = Subtract(x=w412, y=w411) -> (x-y=w405:dbl)
    n296 = Subtract(x=w409, y=w410) -> (x-y=w404:dbl)
    n297 = Index Array "Index Array"(array=w418, index=0) -> (element=w429:i32)
    n298 = Index Array(array=w418, index=1) -> (element=w428:i32)
    n299 = Index Array(array=w418, index=2) -> (element=w425:i32)
    n300 = Divide(x=w429, y=w405) -> (x/y=w424:dbl)
    n301 = Divide(x=w428, y=w404) -> (x/y=w427:dbl)
    n302 = Divide(x=w425, y=w403) -> (x/y=w423:dbl)
    n303 = Compound Arithmetic op=ADD(w424, w427, w423) -> (w422:dbl)
    "Raw data" <- w422
    n304 = Multiply(x=w422, y="he so calib") -> (x*y=w420:dbl)
    n305 = Subtract(x=w420, y="zero") -> (x-y=w393:dbl)
    "Fine Data" <- w393
    n306 = feedback #9(dbl[] []) -> (w414:dbl[])
    n307 = case shown="False" "Start measurement" {
      tunnel: w393 -> [_ w454]
      tunnel: [dbl[] [] w453] -> w415
      tunnel: w414 -> [w440 w452]
      frame False {
        n308 = Array Size(array=w440) -> (size(s)=w441:i32)
        n309 = case shown="10.." w441 {
          selector: w441 -> [_ w450]
          tunnel: w440 -> [_ w449]
          frame 0, Default {
          }
          frame 10.. {
            n310 = Array Subset "Array Subset"(array=w449, index=0) -> (w447:dbl[])  [unwired: 1 in]
            n311 = Add Array Elements(numeric array=w447) -> (sum=w451:dbl)
            n312 = Array Size(array=w447) -> (size(s)=w443:i32)
            n313 = Divide(x=w451, y=w443) -> (x/y=w446:dbl)
            n314 = Multiply(x=w446, y=1000.0) -> (x*y=→"Measurement\nValue":dbl)
            "size array" <- w450
          }
        }
      }
      frame True {
        n315 = Build Array (concatenate) "Build Array"(w452, w454) -> (w453:dbl[])
      }
    }
    n316 = feedback-in #9(w415) -> ()
    n317 = local read "STOP"() -> (w396:bool)
    n318 = call <vilib>:"Mean PtByPt.vi"("x"=w393, "sample length"="sample length", "initialize"="Reset model") -> ("mean"=w394:dbl)  [unwired: 1 in, 1 out]
    n319 = Bundle(w424, w427, w423, "mean"=w394, w393) -> (→"Processing Chart":cluster{dbl, dbl, dbl, "mean":dbl, dbl})  [unwired: 1 in]
    n320 = local read "notifier out"() -> (w397:refnum<notifier>)
    n321 = Or(x=w435, y=w396) -> (x .or. y?=w413:bool)
    n322 = Send Notification(notification=w393, notifier=w397) -> ()  [unwired: 1 in, 2 out]
  }
  n323 = while {
    stop <- w465 stop-if-true
    n324 = case shown="True" "zero" {
      tunnel: "zero" -> [_ w478]
      tunnel: [w467 _] -> w465
      frame False {
        n325 = local read "notifier out"() -> (w468:refnum<notifier>)
        n326 = Get Notifier Status(notifier=w468) -> (error out=w467:errorcluster)  [unwired: 1 in, 4 out]
      }
      frame True {
        n327 = for {
          N: "No. model\nto Zero" -> [_]
          tunnel: w478 -> [_]
          tunnel: [FALSE ("zero")] -> w477
          tunnel: [w480] -> w473 mode=indexing
          tunnel: [w479] -> w471
          i -> [w479]
          n328 = local read "notifier out"() -> (w483:refnum<notifier>)
          n329 = Wait on Notification(notifier=w483, ignore previous (F)=TRUE) -> (notification=w480:dbl)  [unwired: 2 in, 3 out]
        }
        n330 = Increment(x=w471) -> (x+1=w470:i32)
        n331 = Add Array Elements(numeric array=w473) -> (sum=w472:dbl)
        n332 = local write "zero"(w477) -> ()
        n333 = Divide(x=w472, y=w470) -> (x/y=w469:dbl)
        n334 = local read "zero"() -> (w475:dbl)
        n335 = Add(x=w469, y=w475) -> (x+y=w474:dbl)
        n336 = local write "zero"(w474) -> ()
      }
    }
  }
  n337 = call "IMAQ Dispose"("Image"=w5) -> ("error out"=w6:errorcluster)  [unwired: 5 in]
  n338 = call <vilib>:"General Error Handler.vi"("error in (no error)"=w6) -> ()  [unwired: 10 in, 5 out]
  n339 = VISA Close(VISA resource name=w18, error in (no error)=w19) -> (error out=w20:errorcluster)
  n340 = Release Notifier(notifier=w7) -> ()  [unwired: 2 in, 3 out]
  n341 = call <vilib>:"Simple Error Handler.vi"("error in (no error)"=w20) -> ()  [unwired: 1 in, 8 out]
  n342 = call <vilib>:"Close.vi"("Error In"=w4, "LINX Resource"=w3) -> ()  [unwired: 9 in, 1 out]
